vi "ULx Convert 1D Digital Waveform.vi"(0 "task in":refnum<k24>, 7 "data":digitalwaveform[](array[waveform]), 11 "error in":errorcluster) -> (4 "data List":refnum<k24>, 15 "error out":errorcluster)   [LabVIEW 2020]
uses:
  C:/Users/William/Documents/LV 2020 builds/LeaktestDAQ/Source-v33/ULx_LV.dll
  ULx_LV.dll
panel:
  # "channel"
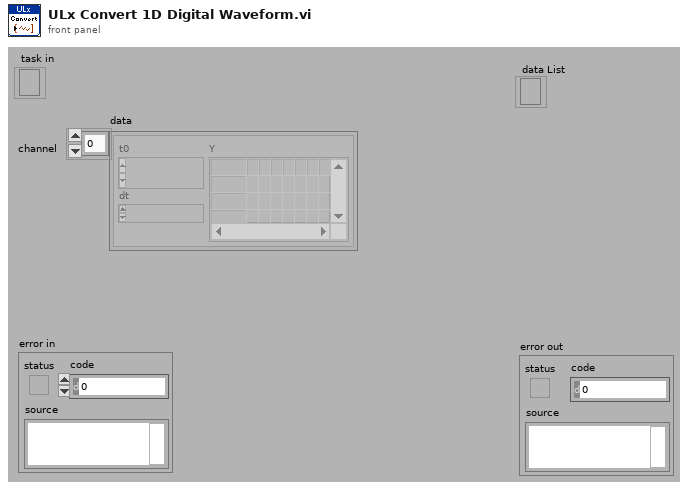
[diagram p1: front panel]
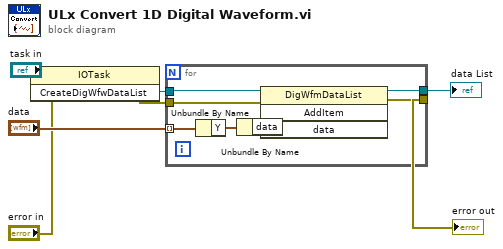
[diagram p0: block diagram]
diagram:
  n1 = invoke class="IOTask" method="CreateDigWfwDataList"(reference="task in", error in="error in") -> (error out=w2:errorcluster, "CreateDigWfwDataList"=w5:refnum<k24>)  [unwired: 1 in, 1 out]
  n2 = for {
    tunnel: "data" -> [w13] mode=indexing
    tunnel: w5 -> [w14]
    tunnel: [w10] -> w4
    tunnel: w2 -> [w9]
    tunnel: [w8] -> w1
    n3 = Unbundle By Name(w13) -> ("Y"=w12:digitaldata)
    n4 = Unbundle By Name(w12) -> ("data"=w11:u8[][])
    n5 = invoke class="DigWfmDataList" method="AddItem"(reference=w14, error in=w9, "data"=w11) -> (reference out=w10:refnum<k24>, error out=w8:errorcluster)  [unwired: 1 in, 2 out]
  }
  "data List" <- w4
  "error out" <- w1
